vi "Trigger Controls.vi"() -> ()   [LabVIEW 2012]
uses:
  Type Defs/Final Output.ctl
  Type Defs/Output Switches.ctl
  Type Defs/Output Values.ctl
panel:
  out "Final Output":T1
  in  "Set Point Alt":dbl=8000.0 min=0.0 max=10000.0 step=1.0
  out "Force Output":T1
  out "Loops":i32=1
  in  "Stop Button":bool
  in  "Tab Control":enum32{"CO2", "AD"}(tab)=enum."AD"
  in  "High CO2 Forces":T2={"A-1, 1"=TRUE, "A-3, 2"=TRUE, "A-4, 3"=FALSE, "A-5, 4"=TRUE, "ABCD-7, 5"=FALSE, "A-8, 6"=TRUE, "B-1,  7"=TRUE, "B-3, 8"=FALSE, "B-4, 9"=TRUE, "B-5, 10"=TRUE, "B-8,  11"=TRUE, "C-1, 12"=TRUE, "C-3, 13"=TRUE, "C-4,  14"=FALSE, "C-5,  15"=TRUE, "C-8, 16"=TRUE, "D-1, 17"=TRUE, "D-3, 18"=TRUE, "D-4, 19"=TRUE, "D-5,  20"=TRUE, "D-8,  21"=TRUE}
  in  "Run C1":T3={"A-1,  1"=inf, "A-3,  2"=inf, "A-4, 3"=9000.0, "A-5, 4"=3400.0, "ABCD-7, 5"=9000.0, "A-8, 6"=8800.0, "B-1,  7"=8800.0, "B-3, 8"=9600.0, "B-4,  9"=9200.0, "B-5, 10"=3400.0, "B-8, 11"=9200.0, "C-1, 12"=1800.0, "C-3, 13"=1800.0, "C-4, 14"=9000.0, "C-5,  15"=8800.0, "C-8, 16"=9200.0, "D-1, 17"=inf, "D-3, 18"=3400.0, "D-4,  19"=1800.0, "D-5,  20"=7000.0, "D-8,  21"=9200.0}
  in  "Run C2":T3={"A-1,  1"=inf, "A-3,  2"=inf, "A-4, 3"=8800.0, "A-5, 4"=3000.0, "ABCD-7, 5"=8800.0, "A-8, 6"=8600.0, "B-1,  7"=8600.0, "B-3, 8"=9600.0, "B-4,  9"=9000.0, "B-5, 10"=3000.0, "B-8, 11"=9000.0, "C-1, 12"=1400.0, "C-3, 13"=1400.0, "C-4, 14"=8800.0, "C-5,  15"=8600.0, "C-8, 16"=9000.0, "D-1, 17"=inf, "D-3, 18"=3000.0, "D-4,  19"=1400.0, "D-5,  20"=6600.0, "D-8,  21"=9000.0}
  in  "Hold C3":T3={"A-1,  1"=1800.0, "A-3,  2"=1800.0, "A-4, 3"=9000.0, "A-5, 4"=3400.0, "ABCD-7, 5"=9000.0, "A-8, 6"=8800.0, "B-1,  7"=8800.0, "B-3, 8"=9600.0, "B-4,  9"=9200.0, "B-5, 10"=3400.0, "B-8, 11"=9200.0, "C-1, 12"=1800.0, "C-3, 13"=1800.0, "C-4, 14"=9000.0, "C-5,  15"=8800.0, "C-8, 16"=9200.0, "D-1, 17"=1800.0, "D-3, 18"=3400.0, "D-4,  19"=1800.0, "D-5,  20"=7000.0, "D-8,  21"=9200.0}
  in  "Hold C4":T3={"A-1,  1"=1400.0, "A-3,  2"=1400.0, "A-4, 3"=8800.0, "A-5, 4"=3000.0, "ABCD-7, 5"=8800.0, "A-8, 6"=8600.0, "B-1,  7"=8600.0, "B-3, 8"=9600.0, "B-4,  9"=9000.0, "B-5, 10"=3000.0, "B-8, 11"=9000.0, "C-1, 12"=1400.0, "C-3, 13"=1400.0, "C-4, 14"=8800.0, "C-5,  15"=8600.0, "C-8, 16"=9000.0, "D-1, 17"=1400.0, "D-3, 18"=3000.0, "D-4,  19"=1400.0, "D-5,  20"=6600.0, "D-8,  21"=9000.0}
  out "Force State":T1
  in  "CO2 ppm":dbl(slide) scale=0.0..10000.0 scale format="%#.0f"
  out "AD State":T1
  out "AD Output":T1
  in  "Hold A4":T3={"A-1,  1"=-150.0, "A-3,  2"=-150.0, "A-4, 3"=-30.0, "A-5, 4"=-250.0, "ABCD-7, 5"=-30.0, "A-8, 6"=inf, "B-1,  7"=inf, "B-3, 8"=80.0, "B-4,  9"=15.0, "B-5, 10"=-250.0, "B-8, 11"=15.0, "C-1, 12"=-300.0, "C-3, 13"=-300.0, "C-4, 14"=-30.0, "C-5,  15"=inf, "C-8, 16"=15.0, "D-1, 17"=-150.0, "D-3, 18"=-250.0, "D-4,  19"=-300.0, "D-5,  20"=-300.0, "D-8,  21"=650.0}
  in  "Hold A3":T3={"A-1,  1"=0.0, "A-3,  2"=0.0, "A-4, 3"=50.0, "A-5, 4"=-150.0, "ABCD-7, 5"=50.0, "A-8, 6"=inf, "B-1,  7"=inf, "B-3, 8"=150.0, "B-4,  9"=60.0, "B-5, 10"=-150.0, "B-8, 11"=60.0, "C-1, 12"=-200.0, "C-3, 13"=-200.0, "C-4, 14"=50.0, "C-5,  15"=inf, "C-8, 16"=60.0, "D-1, 17"=0.0, "D-3, 18"=-150.0, "D-4,  19"=-200.0, "D-5,  20"=-200.0, "D-8,  21"=700.0}
  in  "Run A2":T3={"A-1,  1"=inf, "A-3,  2"=inf, "A-4, 3"=-30.0, "A-5, 4"=-80.0, "ABCD-7, 5"=-30.0, "A-8, 6"=inf, "B-1,  7"=inf, "B-3, 8"=80.0, "B-4,  9"=15.0, "B-5, 10"=-80.0, "B-8, 11"=15.0, "C-1, 12"=-50.0, "C-3, 13"=-50.0, "C-4, 14"=-30.0, "C-5,  15"=inf, "C-8, 16"=15.0, "D-1, 17"=inf, "D-3, 18"=0.0, "D-4,  19"=-50.0, "D-5,  20"=-80.0, "D-8,  21"=650.0}
  in  "High AD Diff":T2={"A-1, 1"=FALSE, "A-3, 2"=FALSE, "A-4, 3"=FALSE, "A-5, 4"=TRUE, "ABCD-7, 5"=FALSE, "A-8, 6"=TRUE, "B-1,  7"=FALSE, "B-3, 8"=FALSE, "B-4, 9"=FALSE, "B-5, 10"=TRUE, "B-8,  11"=TRUE, "C-1, 12"=FALSE, "C-3, 13"=FALSE, "C-4,  14"=FALSE, "C-5,  15"=TRUE, "C-8, 16"=TRUE, "D-1, 17"=FALSE, "D-3, 18"=FALSE, "D-4, 19"=FALSE, "D-5,  20"=FALSE, "D-8,  21"=TRUE}
  in  "Delay S":T3={"A-1,  1"=30.0, "A-3,  2"=30.0, "A-4, 3"=1.0, "A-5, 4"=30.0, "ABCD-7, 5"=1.0, "A-8, 6"=1.0, "B-1,  7"=1.0, "B-3, 8"=1.0, "B-4,  9"=1.0, "B-5, 10"=30.0, "B-8, 11"=1.0, "C-1, 12"=30.0, "C-3, 13"=30.0, "C-4, 14"=1.0, "C-5,  15"=1.0, "C-8, 16"=1.0, "D-1, 17"=30.0, "D-3, 18"=30.0, "D-4,  19"=30.0, "D-5,  20"=30.0, "D-8,  21"=1.0}
  in  "Run A1":T3={"A-1,  1"=inf, "A-3,  2"=inf, "A-4, 3"=50.0, "A-5, 4"=0.0, "ABCD-7, 5"=50.0, "A-8, 6"=inf, "B-1,  7"=inf, "B-3, 8"=150.0, "B-4,  9"=60.0, "B-5, 10"=0.0, "B-8, 11"=60.0, "C-1, 12"=15.0, "C-3, 13"=15.0, "C-4, 14"=50.0, "C-5,  15"=inf, "C-8, 16"=60.0, "D-1, 17"=inf, "D-3, 18"=0.0, "D-4,  19"=15.0, "D-5,  20"=0.0, "D-8,  21"=700.0}
  in  "Alt Dif M":dbl(slide)=1000.0 scale=-1000.0..1000.0
  in  "Set Point Force":T3={"A-1,  1"=inf, "A-3,  2"=inf, "A-4, 3"=inf, "A-5, 4"=inf, "ABCD-7, 5"=inf, "A-8, 6"=inf, "B-1,  7"=inf, "B-3, 8"=inf, "B-4,  9"=inf, "B-5, 10"=inf, "B-8, 11"=inf, "C-1, 12"=inf, "C-3, 13"=inf, "C-4, 14"=inf, "C-5,  15"=inf, "C-8, 16"=inf, "D-1, 17"=inf, "D-3, 18"=inf, "D-4,  19"=inf, "D-5,  20"=6000.0, "D-8,  21"=inf}
  in  "Mode":enum16{"Run", "Hold", "Off"}(ring)=enum."Off"
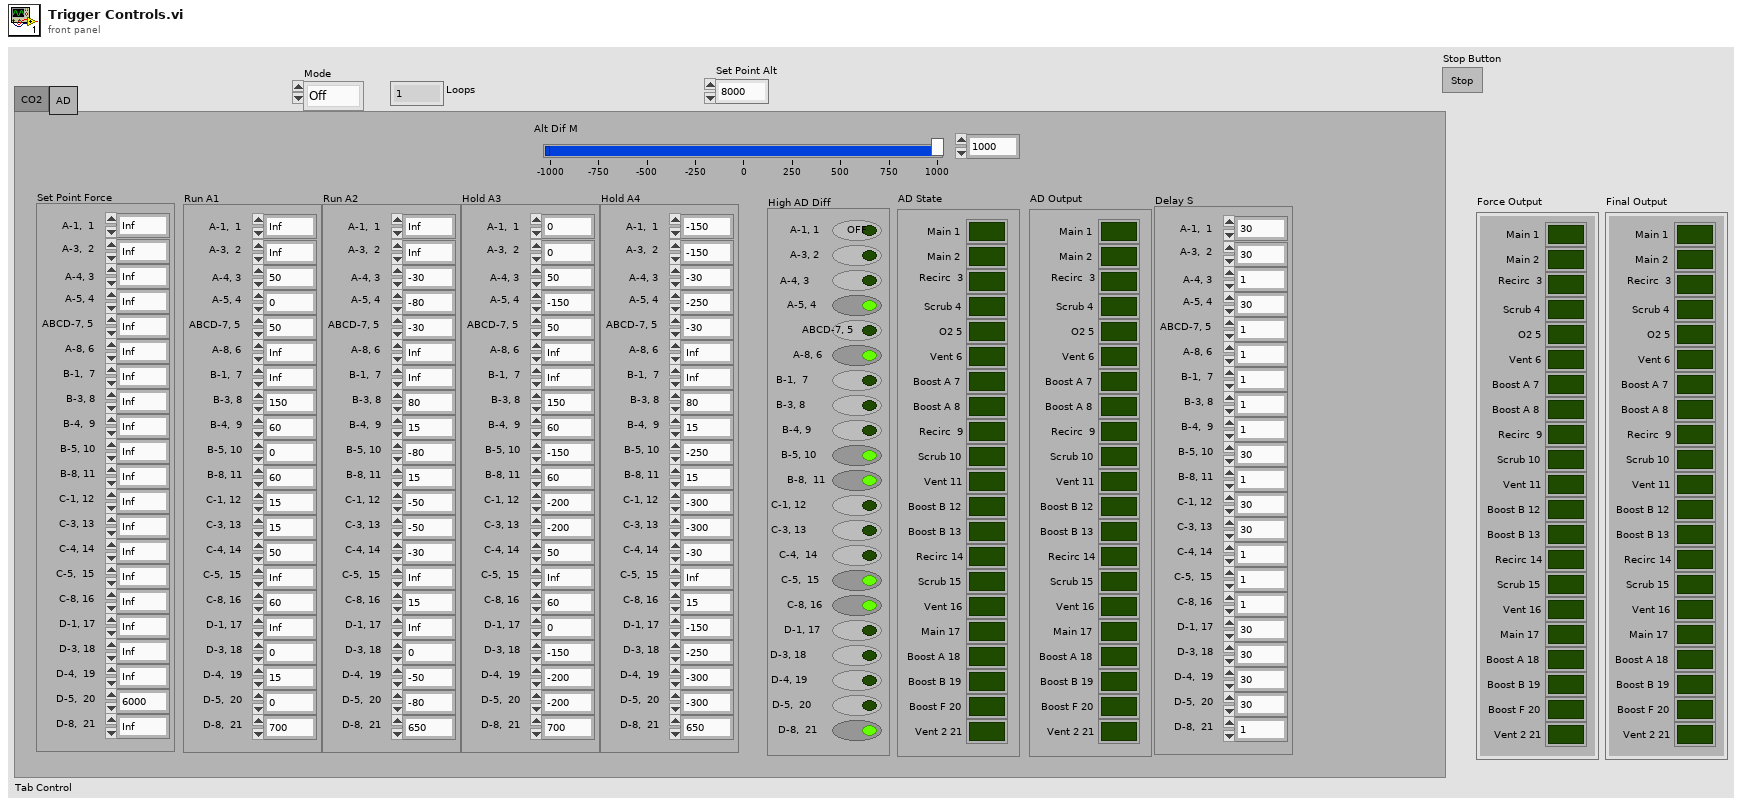
[diagram p1: front panel]
types:
  T1 = typedef "Final Output.ctl" = cluster{"Main 1":bool, "Main 2":bool, "Recirc  3":bool, "Scrub 4":bool, "O2 5":bool, "Vent 6":bool, "Boost A 7":bool, "Boost A 8":bool, "Recirc  9":bool, "Scrub 10":bool, "Vent 11":bool, "Boost B 12":bool, "Boost B 13":bool, "Recirc 14":bool, "Scrub 15":bool, "Vent 16":bool, "Main 17":bool, "Boost A 18":bool, "Boost B 19":bool, "Boost F 20":bool, "Vent 2 21":bool}
  T2 = typedef "Output Switches.ctl" = cluster{"A-1, 1":bool, "A-3, 2":bool, "A-4, 3":bool, "A-5, 4":bool, "ABCD-7, 5":bool, "A-8, 6":bool, "B-1,  7":bool, "B-3, 8":bool, "B-4, 9":bool, "B-5, 10":bool, "B-8,  11":bool, "C-1, 12":bool, "C-3, 13":bool, "C-4,  14":bool, "C-5,  15":bool, "C-8, 16":bool, "D-1, 17":bool, "D-3, 18":bool, "D-4, 19":bool, "D-5,  20":bool, "D-8,  21":bool}
  T3 = typedef "Output Values.ctl" = cluster{"A-1,  1":dbl, "A-3,  2":dbl, "A-4, 3":dbl, "A-5, 4":dbl, "ABCD-7, 5":dbl, "A-8, 6":dbl, "B-1,  7":dbl, "B-3, 8":dbl, "B-4,  9":dbl, "B-5, 10":dbl, "B-8, 11":dbl, "C-1, 12":dbl, "C-3, 13":dbl, "C-4, 14":dbl, "C-5,  15":dbl, "C-8, 16":dbl, "D-1, 17":dbl, "D-3, 18":dbl, "D-4,  19":dbl, "D-5,  20":dbl, "D-8,  21":dbl}
  T4 = cluster{"Main 1":bool, "Main 2":bool, "Recirc  3":bool, "Boost A 7":bool, "Recirc  9":bool, "Scrub 4":bool, "Scrub 10":bool, "O2 5":bool, "Vent 6":bool, "Boost A 8":bool, "Vent 11":bool, "Boost B 12":bool, "Boost B 13":bool, "Recirc 14":bool, "Scrub 15":bool, "Vent 16":bool, "Main 17":bool, "Boost A 18":bool, "Boost B 19":bool, "Boost F 20":bool, "Vent 2 21":bool}
  T5 = cluster{"A-1,  1":bool, "A-3,  2":bool, "A-4, 3":bool, "A-5, 4":bool, "ABCD-7, 5":bool, "A-8, 6":bool, "B-1,  7":bool, "B-3, 8":bool, "B-4,  9":bool, "B-5, 10":bool, "B-8, 11":bool, "C-1, 12":bool, "C-3, 13":bool, "C-4, 14":bool, "C-5,  15":bool, "C-8, 16":bool, "D-1, 17":bool, "D-3, 18":bool, "D-4,  19":bool, "D-5,  20":bool, "D-8,  21":bool}
  T6 = cluster{bool, bool, bool, bool, bool, bool, bool, bool, bool, bool, bool, bool, bool, bool, bool, bool, bool, bool, bool, bool, bool}
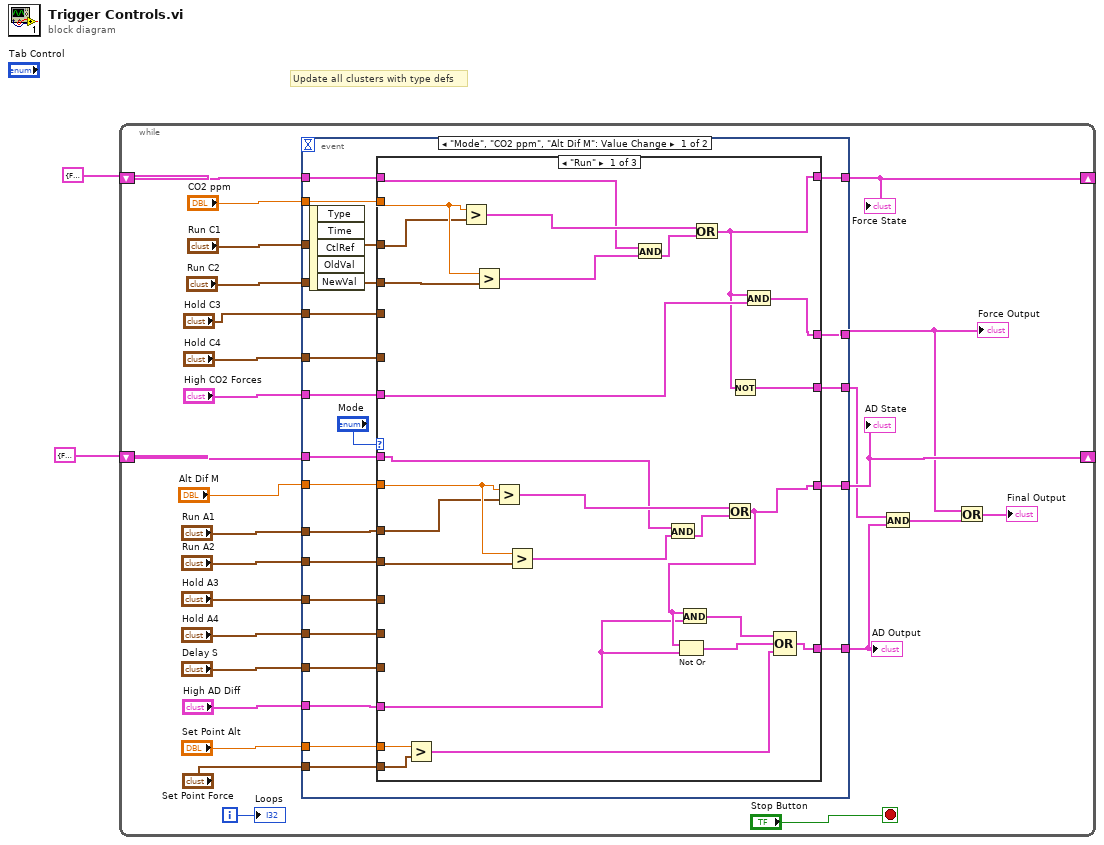
[diagram p0: block diagram]
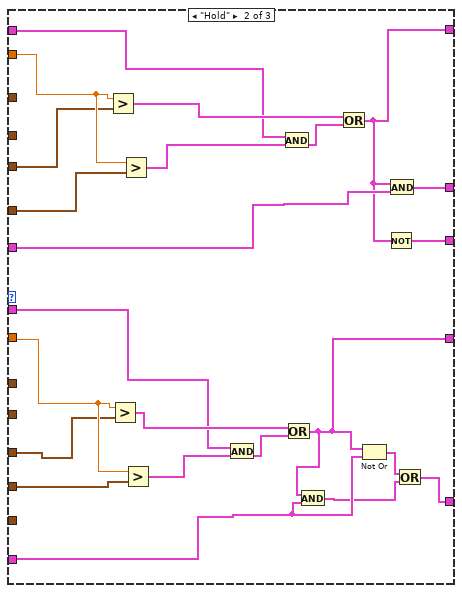
[diagram p2: hidden frame]
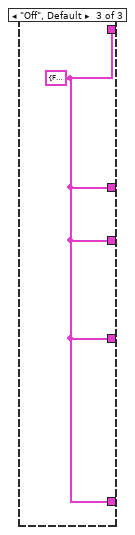
[diagram p3: hidden frame]
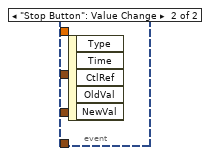
[diagram p4: hidden frame]
diagram:
  # "Update all clusters with type defs"
  n1 = while {
    shift-right: [w23] -> _
    shift-left: T4 {"Main 1"=FALSE, "Main 2"=FALSE, "Recirc  3"=FALSE, "Boost A 7"=FALSE, "Recirc  9"=FALSE, "Scrub 4"=FALSE, "Scrub 10"=FALSE, "O2 5"=FALSE, "Vent 6"=FALSE, "Boost A 8"=FALSE, "Vent 11"=FALSE, "Boost B 12"=FALSE, "Boost B 13"=FALSE, "Recirc 14"=FALSE, "Scrub 15"=FALSE, "Vent 16"=FALSE, "Main 17"=FALSE, "Boost A 18"=FALSE, "Boost B 19"=FALSE, "Boost F 20"=FALSE, "Vent 2 21"=FALSE} -> [w21]
    shift-right: [w11] -> _
    shift-left: T4 {"Main 1"=FALSE, "Main 2"=FALSE, "Recirc  3"=FALSE, "Boost A 7"=FALSE, "Recirc  9"=FALSE, "Scrub 4"=FALSE, "Scrub 10"=FALSE, "O2 5"=FALSE, "Vent 6"=FALSE, "Boost A 8"=FALSE, "Vent 11"=FALSE, "Boost B 12"=FALSE, "Boost B 13"=FALSE, "Recirc 14"=FALSE, "Scrub 15"=FALSE, "Vent 16"=FALSE, "Main 17"=FALSE, "Boost A 18"=FALSE, "Boost B 19"=FALSE, "Boost F 20"=FALSE, "Vent 2 21"=FALSE} ("AD State") -> [w10]
    i -> [w20]
    stop <- "Stop Button" stop-if-true
    n2 = event shown="[0] \"Mode\", \"CO2 ppm\", \"Alt Dif M\": Value Change" {
      selector: _ -> [_ _]
      dyn-events: _ -> [_ _]
      timeout: _ -> [_ _]
      tunnel: "CO2 ppm" -> [w51 _]
      tunnel: "Run C1" -> [w50 _]
      tunnel: "Run C2" -> [w49 _]
      tunnel: "Hold C3" -> [w48 _]
      tunnel: "Hold C4" -> [w47 _]
      tunnel: [w46 _] -> w23
      tunnel: w21 -> [w45 _]
      tunnel: "High CO2 Forces" -> [w43 _]
      tunnel: [w42 _] -> w7
      tunnel: "Alt Dif M" -> [w41 _]
      tunnel: "Run A1" -> [w40 _]
      tunnel: "Run A2" -> [w39 _]
      tunnel: "Hold A3" -> [w38 _]
      tunnel: "Hold A4" -> [w37 _]
      tunnel: "Delay S" -> [w36 _]
      tunnel: "High AD Diff" -> [w35 _]
      tunnel: [w34 _] -> w11
      tunnel: w10 -> [w33 _]
      tunnel: [w32 _] -> w5
      tunnel: "Set Point Alt" -> [w31 _]
      tunnel: "Set Point Force" -> [w30 _]
      tunnel: [w29 _] -> w4
      event "Mode", "CO2 ppm", "Alt Dif M": Value Change {
        n3 = event-data() -> ()  [unwired: 1 in, 5 out]
        n4 = case shown="\"Run\"" "Mode" {
          tunnel: w51 -> [w76 w97 _]
          tunnel: w50 -> [w75 _ _]
          tunnel: [w53 w81 w101] -> w46
          tunnel: w49 -> [w77 _ _]
          tunnel: w48 -> [_ w96 _]
          tunnel: w47 -> [_ w95 _]
          tunnel: w45 -> [w72 w98 _]
          tunnel: w43 -> [w54 w87 _]
          tunnel: [w63 w88 w101] -> w42
          tunnel: w41 -> [w68 w92 _]
          tunnel: w40 -> [w67 _ _]
          tunnel: w39 -> [w66 _ _]
          tunnel: w38 -> [_ w79 _]
          tunnel: w37 -> [_ w78 _]
          tunnel: w36 -> [_ _ _]
          tunnel: w35 -> [w61 w85 _]
          tunnel: [w62 w86 w101] -> w34
          tunnel: w33 -> [w69 w91 _]
          tunnel: [w55 w82 w101] -> w32
          tunnel: w31 -> [w58 _ _]
          tunnel: w30 -> [w57 _ _]
          tunnel: [w52 w80 w101] -> w29
          frame "Run" {
            n5 = Greater?(x=w58, y=w57) -> (0:w56:T5)
            n6 = Greater?(x=w76, y=w75) -> (0:w74:T5)
            n7 = Greater?(x=w76, y=w77) -> (0:w65:T5)
            n8 = Greater?(x=w68, y=w67) -> (0:w71:T5)
            n9 = Greater?(x=w68, y=w66) -> (0:w64:T5)
            n10 = And(x=w72, y=w65) -> (x .and. y?=w73:T6)
            n11 = And(x=w69, y=w64) -> (x .and. y?=w70:T6)
            n12 = Or(x=w74, y=w73) -> (x .or. y?=w53:T6)
            n13 = Or(x=w71, y=w70) -> (x .or. y?=w62:T6)
            n14 = Not Or(1:w61, 2:w62) -> (0:w59:T2)
            n15 = And(x=w62, y=w61) -> (x .and. y?=w60:T2)
            n16 = Not(x=w53) -> (.not. x?=w52:T6)
            n17 = And(x=w53, y=w54) -> (x .and. y?=w63:T2)
            n18 = Compound Arithmetic op=OR(w60, w59, w56) -> (w55:T2)
          }
          frame "Hold" {
            n19 = Greater?(x=w97, y=w96) -> (0:w100:T5)
            n20 = Greater?(x=w92, y=w79) -> (0:w94:T5)
            n21 = Greater?(x=w97, y=w95) -> (0:w90:T5)
            n22 = Greater?(x=w92, y=w78) -> (0:w89:T5)
            n23 = And(x=w91, y=w89) -> (x .and. y?=w93:T6)
            n24 = And(x=w98, y=w90) -> (x .and. y?=w99:T6)
            n25 = Or(x=w94, y=w93) -> (x .or. y?=w86:T6)
            n26 = And(x=w86, y=w85) -> (x .and. y?=w83:T2)
            n27 = Or(x=w100, y=w99) -> (x .or. y?=w81:T6)
            n28 = Not Or(1:w85, 2:w86) -> (0:w84:T2)
            n29 = Not(x=w81) -> (.not. x?=w80:T6)
            n30 = And(x=w81, y=w87) -> (x .and. y?=w88:T2)
            n31 = Or(x=w84, y=w83) -> (x .or. y?=w82:T2)
          }
          frame "Off", Default {
            w101 = T4 {"Main 1"=FALSE, "Main 2"=FALSE, "Recirc  3"=FALSE, "Boost A 7"=FALSE, "Recirc  9"=FALSE, "Scrub 4"=FALSE, "Scrub 10"=FALSE, "O2 5"=FALSE, "Vent 6"=FALSE, "Boost A 8"=FALSE, "Vent 11"=FALSE, "Boost B 12"=FALSE, "Boost B 13"=FALSE, "Recirc 14"=FALSE, "Scrub 15"=FALSE, "Vent 16"=FALSE, "Main 17"=FALSE, "Boost A 18"=FALSE, "Boost B 19"=FALSE, "Boost F 20"=FALSE, "Vent 2 21"=FALSE}
          }
        }
      }
      event "Stop Button": Value Change {
        n32 = event-data() -> ()  [unwired: 1 in, 5 out]
      }
    }
    "Force State" <- w23
    "Force Output" <- w7
    "AD State" <- w11
    "AD Output" <- w5
    n33 = And(x=w4, y=w5) -> (x .and. y?=w3:T2)
    n34 = Or(x=w7, y=w3) -> (x .or. y?=→"Final Output":T2)
    "Loops" <- w20
  }
